vi "speedmeasure.vi"() -> ()   [LabVIEW 2013]
uses:
  <vilib>/Analysis/3filter.llb/Filter Passband Type.ctl
  <vilib>/Instr/_visa.llb/VISA Configure Serial Port (Instr).vi
  <vilib>/ptbypt/NI_PtbyPt.lvlib
  <vilib>/Analysis/NI_AALBase.lvlib
panel:
  in  "stop 2":bool
  in  "Slide":dbl(slide) scale=0.0..5.0
  out "Gauge":dbl(knob) scale=0.0..5.0
  in  "stop":bool
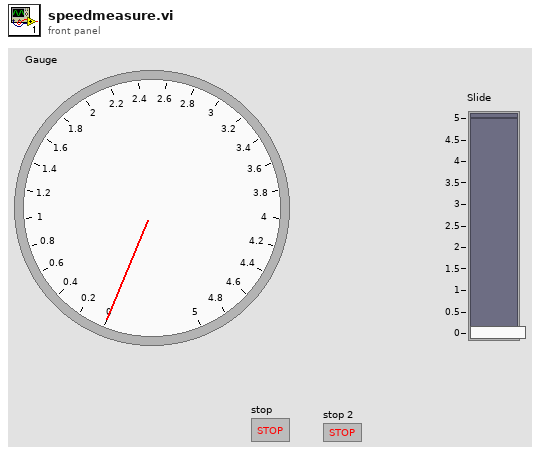
[diagram p1: front panel]
types:
  T1 = typedef "NI_AALBase.lvlib/Filter Passband Type.ctl" = enum32{"Lowpass", "Highpass", "Bandpass", "Bandstop"}
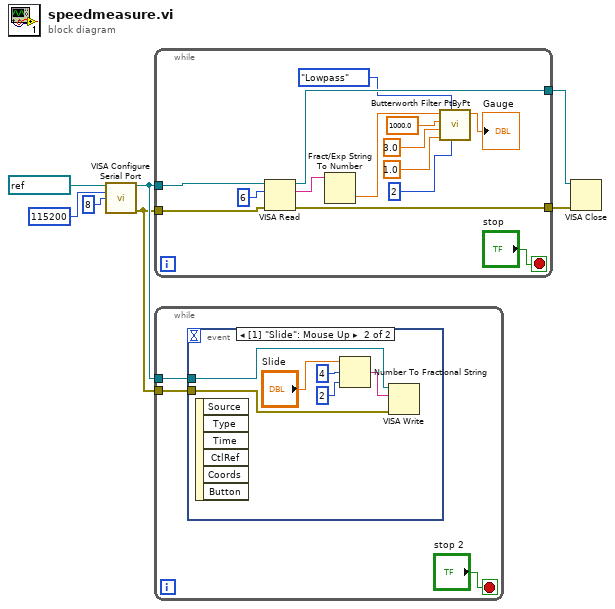
[diagram p0: block diagram]
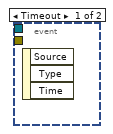
[diagram p2: hidden frame]
diagram:
  n1 = call-poly "VISA Configure Serial Port"("VISA resource name"=refnum<visa-resource-name> "COM7", "baud rate (9600)"=u32 115200, "data bits (8)"=u16 8) -> ("VISA resource name out"=w2:refnum<visa-resource-name>, "error out"=w1:errorcluster)  [unwired: 11 in]
  n2 = while {
    tunnel: w2 -> [w20]
    tunnel: w1 -> [w16]
    tunnel: [w19] -> w5
    tunnel: [w18] -> w4
    stop <- "stop" stop-if-true
    n3 = VISA Read(VISA resource name=w20, byte count=u32 6, error in (no error)=w16) -> (VISA resource name out=w19:refnum<visa-resource-name>, read buffer=w15:string, error out=w18:errorcluster)  [unwired: 1 out]
    n4 = Fract/Exp String To Number(string=w15) -> (number=w13:dbl)  [unwired: 3 in, 1 out]
    n5 = call <vilib>:"Butterworth Filter PtByPt.vi"("order"=2, "filter type"=Filter_Passband_Type."Lowpass", "low cutoff freq: fl"=1.0, "high cutoff freq: fh"=3.0, "sampling freq: fs"=1000.0, "x"=w13) -> ("Filtered x"=→"Gauge":dbl)  [unwired: 3 in, 1 out]
  }
  n6 = while {
    tunnel: w2 -> [w24]
    tunnel: w1 -> [w23]
    stop <- "stop 2" stop-if-true
    n7 = event shown="[1] \"Slide\": Mouse Up" {
      selector: _ -> [_ _]
      dyn-events: _ -> [_ _]
      timeout: _ -> [_ _]
      tunnel: w24 -> [_ w27]
      tunnel: w23 -> [_ w26]
      event Timeout {
        n8 = event-data() -> ()  [unwired: 1 in, 3 out]
      }
      event "Slide": Mouse Up {
        n9 = event-data() -> ()  [unwired: 1 in, 6 out]
        n10 = Number To Fractional String(number="Slide", width (-)=i16 4, precision (6)=i16 2) -> (F-format string=w28:string)  [unwired: 1 in]
        n11 = VISA Write(VISA resource name=w27, write buffer=w28, error in (no error)=w26) -> ()  [unwired: 3 out]
      }
    }
  }
  n12 = VISA Close(VISA resource name=w5, error in (no error)=w4) -> ()  [unwired: 1 out]
